vi "Inputs Array Save Log File.vi"(7 "Status?":string, 8 "loop counters":i32, 9 "Inputs String Array":string[](array[string]), 10 "filename":string="C:\\LILP_log.txt", 11 "Input channel number(ex:1 2 3 ...Max5)":string="3") -> ()   [LabVIEW 2011]
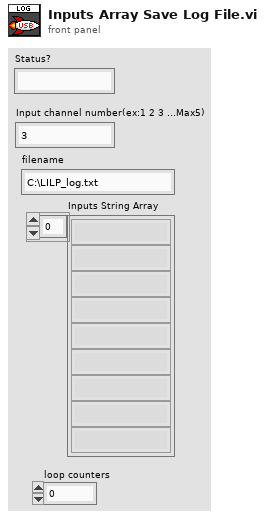
[diagram p1: front panel]
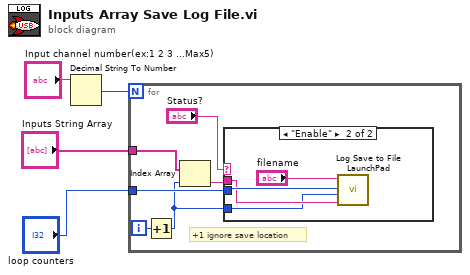
[diagram p0: block diagram]
diagram:
  n1 = Decimal String To Number(string="Input channel number(ex:1 2 3 ...Max5)") -> (number=w2:i32)  [unwired: 2 in, 1 out]
  n2 = for {
    N: w2 -> [_]
    tunnel: "Inputs String Array" -> [w10]
    tunnel: "loop counters" -> [w9]
    i -> [w6]
    # "+1 ignore save location"
    n3 = Increment(x=w6) -> (x+1=w5:i32)
    n4 = Index Array(array=w10, index=w5) -> (element=w8:string)
    n5 = case shown="\"Enable\"" "Status?" {
      tunnel: w8 -> [_ w12]
      tunnel: w9 -> [_ w13]
      tunnel: w5 -> [_ w11]
      frame "Disable", Default {
      }
      frame "Enable" {
        n6 = call "Log Save to File LaunchPad.vi"("data"=w12, "datastream ID"=w11, "cycle"=w13, "filename"="filename") -> ()  [unwired: 8 in]
      }
    }
  }
